vi "channel_conf_ASIC_2.vi"(0 "connection ID":refnum<k5>, 1 "Ring":u16(ring)=4 items=["Channel 0", "Channel 1", "Channel 2", "Channel 3", "Channel 4", "Channel 5", "Channel 6"], 5 "Id in":u32, 7 "Clip_sel_b":u32=2, 9 "CompBuf_en_b":bool, 11 "error out":errorcluster, 12 "Att gain":u32=7, 13 "Ib_ClipVb":u32=20, 14 "Clip_en_b":bool, 15 "Att_en_b":bool) -> (3 "Id out":i32=72, 4 "connection ID out":refnum<k5>, 6 "data read value":u32=72, 8 "written data":u32=72, 10 "error out 2":errorcluster)   [LabVIEW 2012]
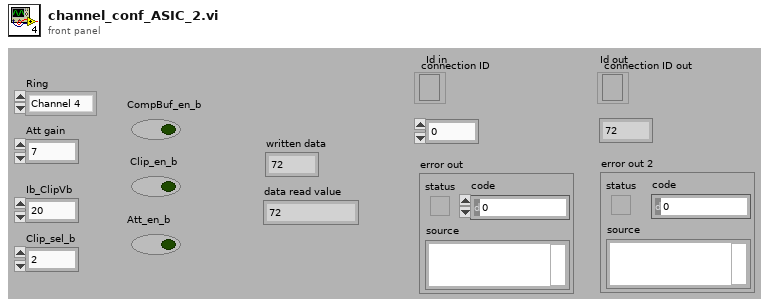
[diagram p1: front panel]
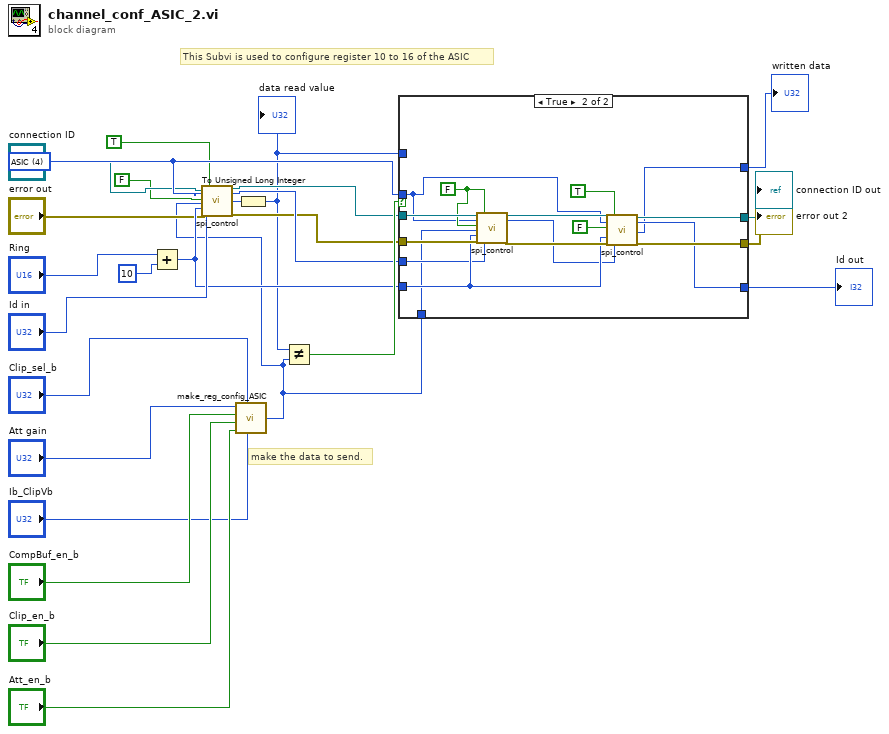
[diagram p0: block diagram]
diagram:
  w16 = u16 4 items=["Attenuation", "Clipping", "Enable channel", "Delay line", "ASIC"] ("Device")
  # "make the data to send."
  # "This Subvi is used to configure register 10 to 16 of the ASIC"
  n1 = Add(x="Ring", y=10 ("Data")) -> (x+y=w17:i32)
  n2 = call "make_reg_config_ASIC.vi"("Ib_ClipVb"="Ib_ClipVb", "Clip_sel_b"="Clip_sel_b", "Att_en_b"="Att_en_b", "Clip_en_b"="Clip_en_b", "CompBuf_en_b"="CompBuf_en_b", "Att gain"="Att gain") -> ("Out reg value"=w1:u32)
  n3 = call "spi_control.vi"("connection ID"="connection ID", "Device"=w16, "Read/#write"=FALSE, "Data"=w1, "Register or channel"=w17, "error in"="error out", "Read physical"=TRUE, "Id in"="Id in") -> ("connection ID out"=w10:refnum<k5>, "Id out"=w18:i32, "data read value"=w7:u32, "error out 2"=w11:errorcluster)  [unwired: 4 in, 4 out]
  n4 = To Unsigned Long Integer(number=w7) -> (unsigned 32bit integer=w2:u32)
  "data read value" <- w2
  n5 = Not Equal?(x=w2, y=w1) -> (x != y?=w25:bool)
  n6 = case shown="True" w25 {
    tunnel: w10 -> [w29 w46]
    tunnel: w11 -> [w30 w45]
    tunnel: [w30 w42] -> w12
    tunnel: [w29 w41] -> w13
    tunnel: w16 -> [_ w39]
    tunnel: w17 -> [_ w36]
    tunnel: w18 -> [w28 w34]
    tunnel: w1 -> [_ w33]
    tunnel: [w28 w32] -> w4
    tunnel: [w27 w31] -> w3
    tunnel: w2 -> [w27 _]
    frame False {
    }
    frame True {
      w40 = FALSE ("Read physical")
      n7 = call "spi_control.vi"("connection ID"=w46, "Device"=w39, "Read/#write"=w40, "Data"=w33, "Register or channel"=w36, "error in"=w45, "Read physical"=w40, "Id in"=w34) -> ("connection ID out"=w44:refnum<k5>, "Id out"=w35:i32, "error out 2"=w43:errorcluster)  [unwired: 4 in, 5 out]
      n8 = call "spi_control.vi"("connection ID"=w44, "Device"=w39, "Read/#write"=FALSE, "Register or channel"=w36, "error in"=w43, "Read physical"=TRUE, "Id in"=w35) -> ("connection ID out"=w41:refnum<k5>, "Id out"=w32:i32, "data read value"=w31:u32, "error out 2"=w42:errorcluster)  [unwired: 5 in, 4 out]
    }
  }
  "connection ID out" <- w13
  "error out 2" <- w12
  "Id out" <- w4
  "written data" <- w3
